vi "SearchUSB_CF.vi"(8 "error in":errorcluster, 10 "USB":string) -> (0 "error out":errorcluster, 2 "USBPort":refnum<visa-resource-name>)   [LabVIEW 2013]
uses:
  <vilib>/registry/registry.llb/Registry SAM.ctl
  <vilib>/registry/registry.llb/Registry RtKey.ctl
  <vilib>/registry/registry.llb/Read Registry Value Simple STR.vi
panel:
  out "为空？":bool
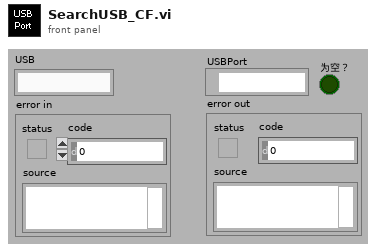
[diagram p1: front panel]
types:
  T1 = cluster{"numSubKeys":i32, "maxSubKeyLen":i32, "maxSubKeyClassLen":i32}
  T2 = typedef "Registry RtKey.ctl" = enum32{"HKEY_CLASSES_ROOT", "HKEY_CURRENT_USER", "HKEY_LOCAL_MACHINE", "HKEY_USERS", "HKEY_PERFORMANCE_DATA", "HKEY_CURRENT_CONFIG", "HKEY_DYN_DATA"}
  T3 = typedef "Registry SAM.ctl" = enum32{"KEY_QUERY_VALUE", "KEY_SET_VALUE", "KEY_CREATE_SUB_KEY", "KEY_ENUMERATE_SUB_KEYS", "KEY_NOTIFY", "KEY_CREATE_LINK", "KEY_READ", "KEY_WRITE", "KEY_ALL_ACCESS", "KEY_READ | KEY_WRITE"}
  T4 = typedef "Registry refnum.ctl" = refnum<k1>
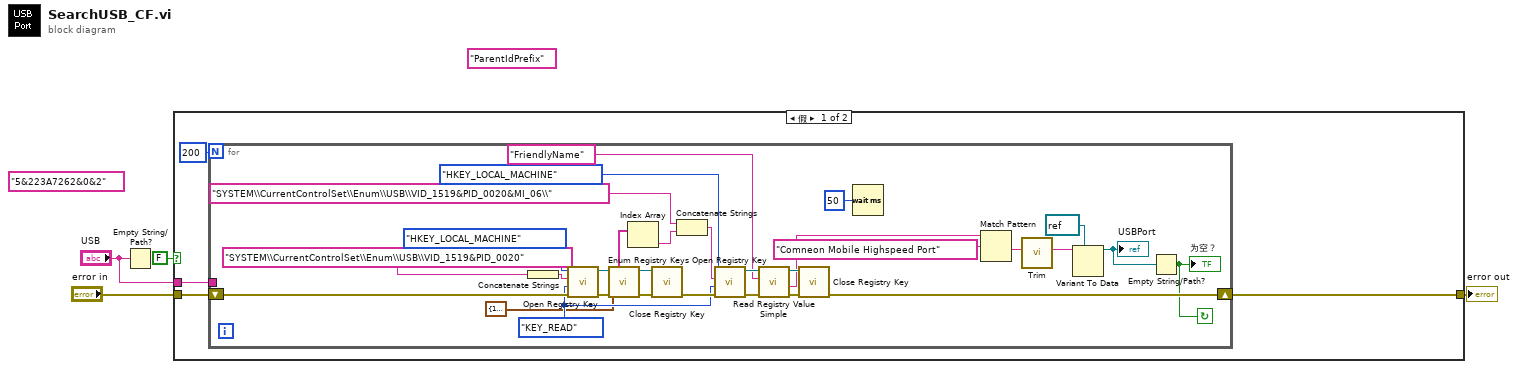
[diagram p0: block diagram]
diagram:
  (unwired) "ParentIdPrefix" ("value")
  (unwired) "5&223A7262&0&2" ("正则表达式")
  n1 = Empty String/Path?(string/path="USB") -> ()  [unwired: 1 out]
  n2 = case shown="假" FALSE {
    tunnel: "error in" -> [w8 w39]
    tunnel: [w6 w39] -> w4
    tunnel: "USB" -> [w7 _]
    frame False {
      n3 = for {
        N: 200 -> [_]
        tunnel: w7 -> [_]
        shift-right: [w26] -> w6
        shift-left: w8 -> [w35]
        stop <- w17 continue-if-true
        w22 = Registry_SAM."KEY_READ" ("security access mask (KEY_READ | KEY_WRITE)")
        n4 = Concatenate Strings("SYSTEM\\CurrentControlSet\\Enum\\USB\\VID_1519&PID_0020" ("subkey")) -> (w37:string)
        n5 = call <vilib>:"Open Registry Key.vi"("error in (no error)"=w35, "security access mask (KEY_READ | KEY_WRITE)"=w22, "subkey"=w37, "root key (HKEY_LOCAL_MACHINE)"=Registry_RtKey."HKEY_LOCAL_MACHINE") -> ("error out"=w15:errorcluster, "refnum out"=w14:T4)  [unwired: 6 out]
        n6 = call <vilib>:"Enum Registry Keys.vi"("error in (no error)"=w15, "subkey info"=T1 {"numSubKeys"=1, "maxSubKeyLen"=15, "maxSubKeyClassLen"=15}, "refnum"=w14) -> ("error out"=w12:errorcluster, "subkeys"=w10:string[], "refnum out"=w13:T4)  [unwired: 6 in]
        n7 = Index Array(array=w10) -> (element=w9:string)  [unwired: 1 in]
        n8 = call <vilib>:"Close Registry Key.vi"("error in (no error)"=w12, "refnum"=w13) -> ("error out"=w27:errorcluster)  [unwired: 5 out]
        n9 = Concatenate Strings("SYSTEM\\CurrentControlSet\\Enum\\USB\\VID_1519&PID_0020&MI_06\\" ("subkey"), w9) -> (w28:string)
        n10 = call <vilib>:"Open Registry Key.vi"("error in (no error)"=w27, "security access mask (KEY_READ | KEY_WRITE)"=w22, "subkey"=w28, "root key (HKEY_LOCAL_MACHINE)"=Registry_RtKey."HKEY_LOCAL_MACHINE") -> ("error out"=w32:errorcluster, "refnum out"=w33:T4)  [unwired: 6 out]
        n11 = call-poly <vilib>:"Read Registry Value Simple.vi"("error in (no error)"=w32, "value"="FriendlyName", "refnum"=w33) -> ("error out"=w30:errorcluster, "String/Binary data"=w24:string, "refnum out"=w34:T4)  [unwired: 1 in, 3 out]
        n12 = call <vilib>:"Close Registry Key.vi"("error in (no error)"=w30, "refnum"=w34) -> ("error out"=w26:errorcluster)  [unwired: 5 out]
        n13 = Wait (ms)(milliseconds to wait=u32 50 ("等待时间（毫秒）")) -> ()  [unwired: 1 out]
        n14 = Match Pattern(string=w24, regular expression="Comneon Mobile Highspeed Port" ("正则表达式")) -> (after substring=w18:string)  [unwired: 4 out]
        n15 = call "Trim.vi"("String"=w18) -> ("TrimStr"=w20:string)  [unwired: 10 in]
        n16 = Variant To Data(type=refnum<visa-resource-name> refnum ("VISA resource name"), Variant=w20) -> (data=w19:refnum<visa-resource-name>)  [unwired: 1 in, 1 out]
        "USBPort" <- w19
        n17 = Empty String/Path?(string/path=w19) -> (empty?=w17:bool)
        "为空？" <- w17
      }
    }
    frame True {
    }
  }
  "error out" <- w4
